vi "启动采配水清洗 (子VI).vi"() -> (0 "error out":T1={"status"=FALSE, "代码"=4, "source"=""} caption="错误输出" {"代码" items=["执行成功"=1, "执行失败，但不知道原因"=2, "命令请求条件错误"=3, "通讯超时"=4, "系统繁忙不能执行"=5, "系统故障"=6, "没有数据"=100]})   [LabVIEW 2016, in "MB SLAVE.lvlib"]
uses:
  MB SLAVE.lvlib
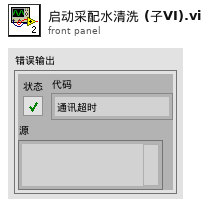
[diagram p1: front panel]
types:
  T1 = cluster{"status":bool, "代码":u16, "source":string}
  T2 = typedef "系统交互.ctl" = cluster{"运行模式":enum16{"维护模式", "常规模式", "应急模式", "质控模式", "性能测试"}, "运行间隔":i16, "流程运行中":bool, "自动运行启动参数":T3, "SYSTEM Interface.总磷总氮类型":enum16{"单模块", "总磷总氮二合一模块", "氨氮总磷二合一模块"}, "多参数运行间隔":i16, "配水时间":dbl, "沉淀时间":dbl, "清洗时间":dbl, "关键参数改变":bool, "温度告警":bool, "湿度告警":bool, "烟感告警":bool, "水浸告警":bool, "开门告警":bool, "超标留样瓶满告警":bool, "SystemTask":enum16{"停机", "待机", "调试", "水样采集", "沉沙", "进样", "仪表测试分析", "反吹", "清洗", "除藻"}, "PumpState":enum16{"--", "只用泵1", "只用泵2", "双泵交替"}, "除藻选择":enum16{"不开除藻", "开除藻"}, "报警信息":enum16{"无报警", "断电报警", "采样管理欠压（源水泵故障）", "进样管路欠压（进样泵/增加泵故障）"}, "软件升级":bool, "固件升级":enum16{"无", "CODMn", "氨氮", "总磷", "总氮", "CODCr"}, "数据传输软件升级":bool, "数采仪软件版本":string}
  T3 = typedef "启动参数.ctl" = cluster{"氨氮":bool, "总磷":bool, "总氮":bool, "多参数":bool, "CODmn":bool, "CODCr":bool, "氟化物":bool, "超标留样":bool, "重金属":bool, "挥发酚":bool, "综合生物毒性":bool}
  T4 = typedef "采配水交互.ctl" = cluster{"测试模式":enum16{"清洗", "开泵X", "开阀X", "关泵X", "关阀X"}, "值":u16}
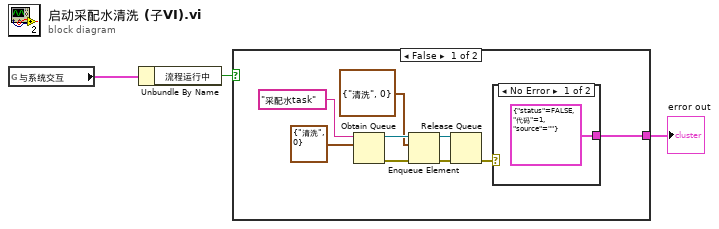
[diagram p0: block diagram]
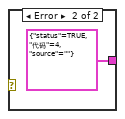
[diagram p2: hidden frame]
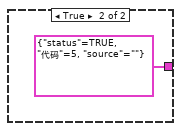
[diagram p3: hidden frame]
diagram:
  n1 = global read "modbus slave全局.vi" "与系统交互"() -> (w2:T2)
  n2 = Unbundle By Name(w2) -> ("流程运行中"=w1:bool)
  n3 = case shown="False" w1 {
    tunnel: [w12 T1 {"status"=TRUE, "代码"=5, "source"=""} ("error out")] -> w3
    frame False {
      n4 = Obtain Queue(name (unnamed)="采配水task" ("名称（未命名）"), element data type=T4 {"测试模式"=enum."清洗", "值"=0} ("测试模式")) -> (queue out=w10:refnum<queue>, error out=w9:errorcluster)  [unwired: 3 in, 1 out]
      n5 = Enqueue Element(queue=w10, element=T4 {"测试模式"=enum."清洗", "值"=0} ("测试模式"), error in (no error)=w9) -> (queue out=w7:refnum<queue>, error out=w8:errorcluster)  [unwired: 1 in, 1 out]
      n6 = Release Queue(queue=w7, error in (no error)=w8) -> (error out=w6:errorcluster)  [unwired: 1 in, 2 out]
      n7 = case shown="No Error" w6 {
        tunnel: [T1 {"status"=FALSE, "代码"=1, "source"=""} ("error out") T1 {"status"=TRUE, "代码"=4, "source"=""} ("error out")] -> w12
        frame No Error {
        }
        frame Error {
        }
      }
    }
    frame True {
    }
  }
  "error out" <- w3
